vi "Dashboard Main.vi"() -> ()   [LabVIEW 2016]
uses:
  <vilib>/Utility/miscctls.llb/LVRowAndColumnTypeDef.ctl
  <vilib>/event_ctls.llb/eventvkey.ctl
  <vilib>/Rock Robotics/Network Tables/NT Read Numeric Array.vi
  <vilib>/Rock Robotics/WPI/Dashboard/WPI_DashboardLogging Global.vi
panel:
  in  "Camera Settings Right":T1={"Frame Rate"=30, "Compression"=30, "Size"=1, "DB Camera Config"=FALSE} {"Frame Rate" scale=1.0..30.0; "Compression" scale=100.0..-1.0; "Size" items=["640x480", "320x240", "160x120"]}
  in  "Camera Name Right":string(combo)="No Camera Selection"
  out "Camera Info":cluster{"Mbps LED":bool, "Mbps":dbl, "fps":dbl} {"fps" format="%#.1g"; "Mbps" format="%#.1g"}
  in  "Camera Settings":T1={"Frame Rate"=30, "Compression"=30, "Size"=1, "DB Camera Config"=FALSE} {"Frame Rate" scale=1.0..30.0; "Compression" scale=100.0..-1.0; "Size" items=["640x480", "320x240", "160x120"]}
  in  "TCP":refnum<k5>
  in  "Rec Mode":enum32{"Stop", "Record", "Playback"}(radio)
  out "Robot IP":string
  out "Image Message":string="Timeout in Camera Communications"
  in  "Dashboard Tab":T2(tab)
  out "Distance (ft)":dbl(slide) scale=1.0..16.25
  in  "Select Auto":string(combo)="Select Autonomous ..."
  out "NT Connection":bool
  out "MotorChart R":cluster{"Numeric":dbl, "Numeric":dbl}(graph)
  out "MotorChart L":cluster{"Numeric":dbl, "Numeric":dbl}(graph)
  out "MotorSliders R":cluster{"MotorSlide1":dbl, "MotorSlide2":dbl} {"MotorSlide2" scale=-1.0..1.0 scale format="%#_2e"; "MotorSlide1" scale=-1.0..1.0 scale format="%#_2e"}
  out "MotorSliders L":cluster{"MotorSlide1":dbl, "MotorSlide2":dbl} {"MotorSlide2" scale=-1.0..1.0 scale format="%#_2e"; "MotorSlide1" scale=-1.0..1.0 scale format="%#_2e"}
  out "JS1 Z":dbl(slide) scale=-1.0..1.0 scale format="%#_2e"
  out "JS1 Graph":cluster{"X":dbl, "Y":dbl}[](graph)
  out "JS1 Buttons":T3
  out "JS2 Z":dbl(slide) scale=-1.0..1.0 scale format="%#_2e"
  out "JS2 Graph":cluster{"X":dbl, "Y":dbl}[](graph)
  out "JS2 Buttons":T3
  out "Mode":T4(ring)=enum."Auto Disabled"
  out "Camera Image Right":T5(plugin-control)
  in  "DB/String 9":string
  in  "DB/String 8":string
  in  "DB/String 7":string
  in  "DB/String 6":string
  in  "DB/String 5":string
  in  "DB/String 4":string
  in  "DB/String 3":string
  in  "DB/String 2":string
  in  "DB/String 1":string
  in  "DB/String 0":string
  in  "DB/Slider 0":dbl(slide) scale=0.0..5.0
  in  "DB/Slider 1":dbl(slide) scale=0.0..5.0
  in  "DB/Slider 2":dbl(slide) scale=0.0..5.0
  in  "DB/Slider 3":dbl(slide) scale=0.0..5.0
  out "DB/LED 3":bool
  out "DB/LED 2":bool
  out "DB/LED 1":bool
  out "DB/LED 0":bool
  in  "DB/Button 3":bool
  in  "DB/Button 2":bool
  in  "DB/Button 1":bool
  in  "DB/Button 0":bool caption="New Name"
  in  "Test Slider":dbl(slide) scale=0.0..100.0 scale format="%#_3g"
  in  "On/Off":bool caption="Solenoid"
  in  "Test Name":u16(ring) items=["Select the test to run..."]
  in  "Test Tree":string(tree)
  in  "Motor":cluster{"Value":dbl, "Enable":bool} {"Value" scale=-1.0..1.0 scale format="%#_3g"}
  out "Progress":T6 {"Test Progress" scale=0.0..100.0}
  in  "Rev/Fwd":cluster{"Forward":bool, "Reverse":bool}
  in  "Test Ring":u16(ring) items=["Monochrome", "Color"]
  out "Cmd Status":string
  in  "Execute Command":bool
  in  "Command Params":string[][](table)
  in  "Command Selection":i32(listbox)
  in  "CheckList":i32(listbox)
  out "Tree":string(tree)
  out "Camera Image":T5(plugin-control)
  out "Background":bool
  in  "Camera Name":string(combo)="No Camera Selection"
  # "HW"
  # "HW"
  # "Joysticks"
  # "Drive Motors"
  # "Front"
  # "Right"
  # "Left"
  # "Back"
  # "This tab is a great place for autonomous settings and robot-specific values.\nPlace controls and indicators inside this tab and match name to\nDashboard Variables on robot. You can also delete this comment."
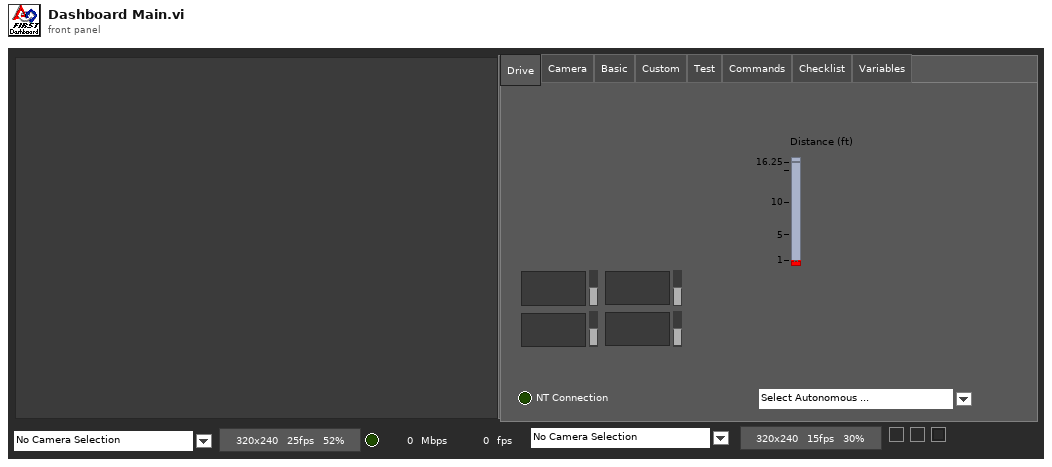
[diagram p1: front panel]
types:
  T1 = cluster{"Frame Rate":i32, "Compression":i32, "Size":u16, "DB Camera Config":bool}
  T2 = enum32{"Drive", "Camera", "Basic", "Custom", "Test", "Commands", "Checklist", "Variables"}
  T3 = cluster{bool, bool, bool, bool, bool, bool, bool, bool, bool, bool, bool, bool}
  T4 = enum8{"Tele-Op Disabled", "Tele-Op Enabled", "Auto Disabled", "Auto Enabled", "Test Disabled", "Test Enabled", "Disconnected", "No Code", "E-Stop"}
  T5 = typedef "IMAQ Image.ctl" = refnum<image>
  T6 = cluster{"Test Progress":u8, "Test Progress Text":string}
  T7 = typedef "Image Type" = u32
  T8 = cluster{"IDs":cluster{"RPC field ID":u16, "Unique ID":u16}, "String":string}
  T9 = enum32{"Drive", "Basic", "Custom", "Test", "Checklist", "Variables"}
  T10 = cluster{"Error Strings":string, "Disable Counts":cluster{u16, u16}, "Rail Faults":cluster{u16, u16, u16}, "Robot IP":string, "DB Mode":u8, "Event Info":cluster{"Name":string, "Type":u8, "Number":u16, "Replay":u8}}
  T11 = cluster{"Storage":cluster{"Disk Free":u64, "RAM Block":u32, "RAM free":u32}, "CPU Utilization":cluster{"CPU % ISR":sgl, "CPU % Time Crit":sgl, "CPU % Timed Str":sgl, "CPU % High":sgl, "CPU % Above":sgl, "CPU % Normal":sgl, "CPU % Low":sgl}, "CAN":cluster{"% Bus Utilization":sgl, "Bus Off Cnt":u32, "TX_FIFO Full Cnt":u32, "Receive Error Cnt":u8, "Transmit Error Cnt":u8}, "HID":cluster{"HID Outputs":u32, "Rumble Low":u16, "Rumble High":u16}[]}
  T12 = cluster{"Status bits":cluster{"Test Mode":bool, "Autonomous":bool, "Enabled":bool, "Code Start":bool, "Brownout":bool, "Reserved 2":bool, "Reserved 3":bool, "E-Stop":bool}, "Code Trace":cluster{"Disabled":bool, "TeleOp":bool, "Auto":bool, "Test":bool}, "Controller Type":enum16{"unknown", "cRIO", "roboRio"}, "Code?":enum16{"unknown", "noCode", "code"}, "Battery V":dbl}
  T13 = cluster{"Control Bits":cluster{"TestMode":bool, "Autonomous":bool, "Enabled":bool, "FMS Present":bool, bool, bool, bool, "E-Stop":bool}, "Team Station ":u8, "Countdown":sgl, "Joystick Values":cluster{"Axes":dbl[], "Buttons":bool[], "POVs":i16[]}[]}
  T14 = cluster{"Axes":dbl[], "Buttons":bool[], "POVs":i16[]}[]
  T15 = cluster{"Axes":dbl[], "Buttons":bool[], "POVs":i16[]}
  T16 = cluster{"Buttons[0]":bool, "Buttons[1]":bool, "Buttons[2]":bool, "Buttons[3]":bool, "Buttons[4]":bool, "Buttons[5]":bool, "Buttons[6]":bool, "Buttons[7]":bool, "Buttons[8]":bool, "Buttons[9]":bool, "Buttons[10]":bool, "Buttons[11]":bool}
  T17 = cluster{"Camera Image":refnum<vi>, "Dashboard Tab":refnum<vi>, "Background":refnum<vi>, "Rec Mode":refnum<vi>, "Test Slider":refnum<vi>, "On/Off ":refnum<vi>, "Test Ring":refnum<vi>, "Rev/Fwd":refnum<vi>, "Test Name":refnum<vi>, "Motor":refnum<vi>, "Progress":refnum<vi>, "CheckList":refnum<vi>, "Tree":refnum<vi>, "Test Tree":refnum<vi>, "Command Params":refnum<vi>, "Command Selection":refnum<vi>, "Execute Command":refnum<vi>, "Cmd Status":refnum<vi>, "Camera Settings":refnum<vi>, "Camera Name":refnum<vi>, "Camera Info":refnum<vi>, "Camera Settings Right":refnum<vi>, "Camera Name Right":refnum<vi>, "Camera Image Right":refnum<vi>}
  T18 = cluster{"Operation":enum16{"Update", "Clear"}, "Color Box":u32}[]
  T19 = typedef "eventvkey.ctl" = enum16{"ASCII", "Enter", "Return", "Shift", "Ctrl", "Alt", "Cmd", "Opt", "Caps", "NumLock", "Clear", "Break", "Up", "Down", "Left", "Right", "Insert", "Delete", "Home", "End", "PageUp", "PageDown", "Escape", "Help", "Pause", "ScrollLock", "F1", "F2", "F3", "F4", "F5", "F6", "F7", "F8", "F9", "F10", "F11", "F12", "F13", "F14", "F15", "F16", "F17", "F18", "F19", "F20", "F21", "F22", "F23", "F24", "Play", "VolumeUp", "VolumeDown", "Mute", "Two Byte Char"}
  T20 = cluster{"Image Size":bool, "Image Type":bool, "Pixel Value":bool, "ROI Information":bool, "Zoom Factor":bool}
  T21 = cluster{"Operation":enum16{"Update", "Clear"}, "Color Box":u32}
  T22 = typedef "LVRowAndColumnTypeDef.ctl" = cluster{"Row":i32, "Column":i32}
  T23 = cluster{"Shift":bool, "Ctrl":bool, "Alt":bool, "Cmd":bool, "Opt":bool}
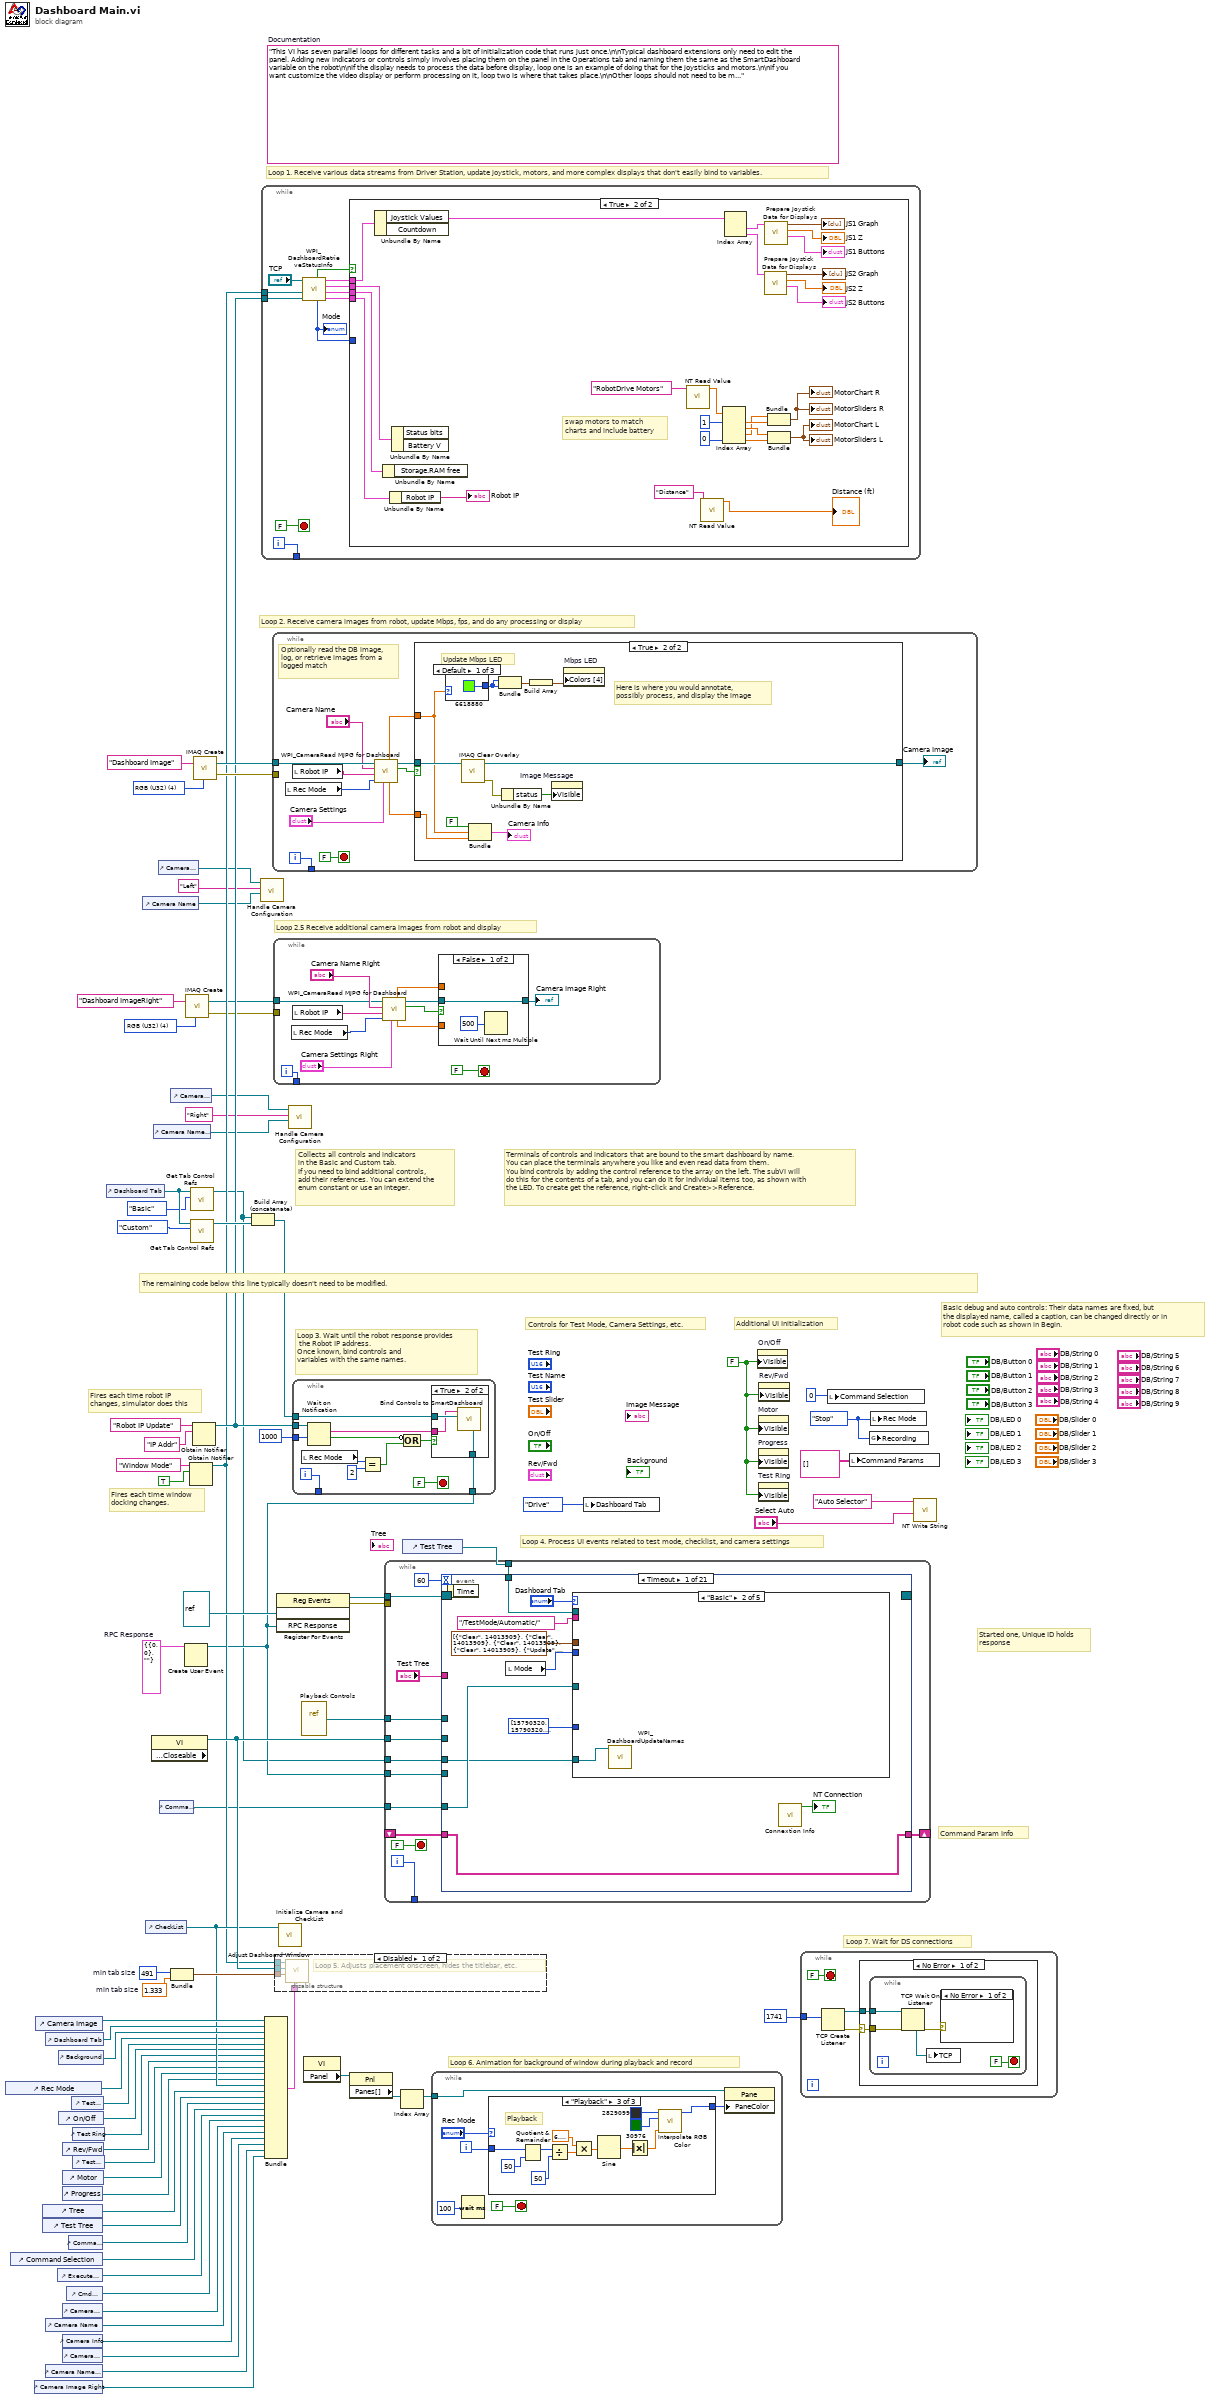
[diagram p0: block diagram]
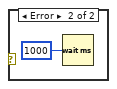
[diagram p4: hidden frame]
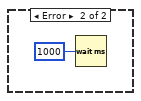
[diagram p5: hidden frame]
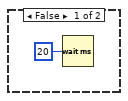
[diagram p6: hidden frame]
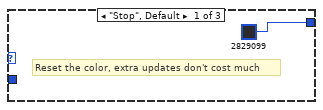
[diagram p7: hidden frame]
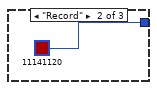
[diagram p8: hidden frame]
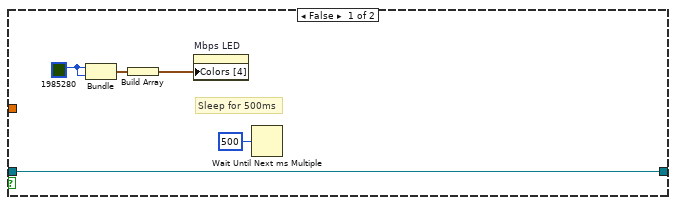
[diagram p10: hidden frame]
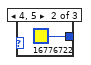
[diagram p11: hidden frame]
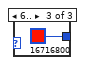
[diagram p12: hidden frame]
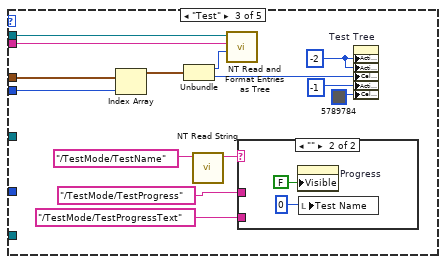
[diagram p14: hidden frame]
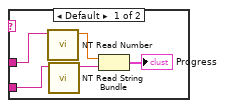
[diagram p15: hidden frame]
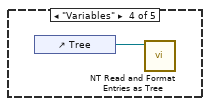
[diagram p16: hidden frame]
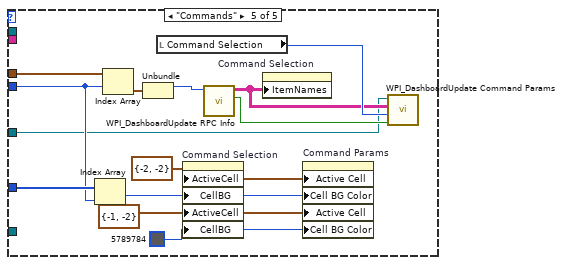
[diagram p17: hidden frame]
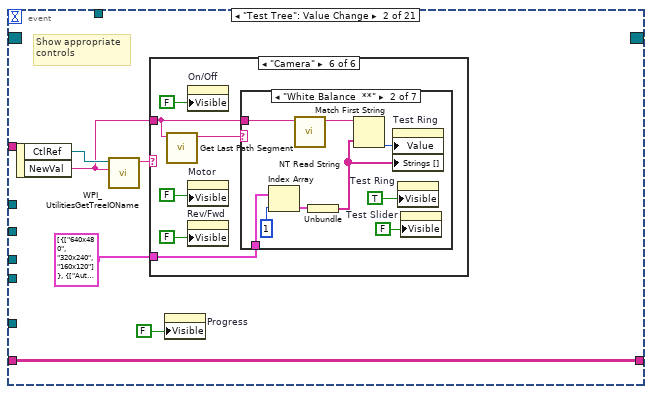
[diagram p18: hidden frame]
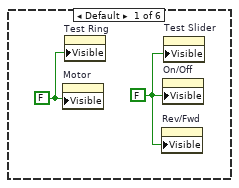
[diagram p19: hidden frame]
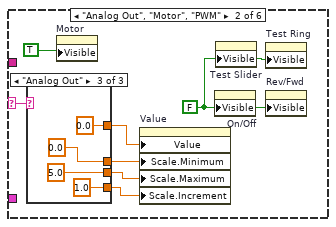
[diagram p20: hidden frame]
diagram:
  w10 = T7 4 items=["Grayscale (U8)", "Grayscale (I16)", "Grayscale (SGL)", "Complex (CSG)", "RGB (U32)", "HSL (U32)", "RGB (U64)"] ("Image Type")
  w26 = T8 {"IDs"={"RPC field ID"=0, "Unique ID"=0}, "String"=""}  # RPC Response
  w51 = 491  # min tab size
  w50 = 1.333  # min tab size
  w58 = enum32{"Stop", "Record", "Playback"}."Stop" ("Rec Mode")
  w33 = FALSE ("Visible")
  (unwired) "This VI has seven parallel loops for different tasks and a bit of initialization code that runs just once.\n\nTypical dashboard extensions only need to edit the panel. Adding new indicators or controls simply involves placing them on the panel in the Operations tab and naming them the same as the SmartDashboard variable on the robot\n\nIf the display needs to process the data before display, loop one is an example of doing that for the joysticks and motors.\n\nIf you want customize the video display or perform processing on it, loop two is where that takes place.\n\nOther loops should not need to be modified. They are pretty standard, and document the task they perform."  # Documentation
  w75 = T7 4 items=["Grayscale (U8)", "Grayscale (I16)", "Grayscale (SGL)", "Complex (CSG)", "RGB (U32)", "HSL (U32)", "RGB (U64)"] ("Image Type")
  # "Loop 2.5 Receive additional camera images from robot and display"
  # "Command Param Info"
  # "Started one, Unique ID holds\nresponse"
  # "Loop 7. Wait for DS connections"
  # "Basic debug and auto controls: Their data names are fixed, but\nthe displayed name, called a caption, can be changed directly or in\nrobot code such as shown in Begin."
  # "Controls for Test Mode, Camera Settings, etc."
  # "Additional UI Initialization"
  # "Loop 6. Animation for background of window during playback and record"
  # "Fires each time robot IP\nchanges, simulator does this"
  # "Fires each time window\ndocking changes."
  # "Collects all controls and indicators\nin the Basic and Custom tab.\nIf you need to bind additional controls,\nadd their references. You can extend the\nenum constant or use an integer."
  # "The remaining code below this line typically doesn't need to be modified."
  # "Loop 4. Process UI events related to test mode, checklist, and camera settings"
  # "Terminals of controls and indicators that are bound to the smart dashboard by name.\nYou can place the terminals anywhere you like and even read data from them.\nYou bind controls by adding the control reference to the array on the left. The subVI will\ndo this for the contents of a tab, and you can do it for individual items too, as shown with\nthe LED. To create get the reference, right-click and Create>>Reference."
  # "Loop 3. Wait until the robot response provides\n the Robot IP address.\nOnce known, bind controls and\nvariables with the same names."
  # "Loop 1. Receive various data streams from Driver Station, update joystick, motors, and more complex displays that don't easily bind to variables."
  # "Loop 2. Receive camera images from robot, update Mbps, fps, and do any processing or display"
  n1 = control-ref of="Rec Mode"() -> (w39:refnum<vi>)
  n2 = control-ref of="Command Selection"() -> (w25:refnum<vi>)
  n3 = control-ref of="Camera Image Right"() -> (w1:refnum<vi>)
  n4 = control-ref of="Camera Image"() -> (w53:refnum<vi>)
  n5 = control-ref of="Tree"() -> (w43:refnum<vi>)
  n6 = control-ref of="Test Tree"() -> (w42:refnum<vi>)
  n7 = control-ref of="Dashboard Tab"() -> (w52:refnum<vi>)
  n8 = control-ref of="Camera Name"() -> (w16:refnum<vi>)
  n9 = control-ref of="Camera Name Right"() -> (w2:refnum<vi>)
  n10 = control-ref of="Execute Command"() -> (w27:refnum<vi>)
  n11 = control-ref of="Background"() -> (w48:refnum<vi>)
  n12 = control-ref of="On/Off"() -> (w37:refnum<vi>)
  n13 = control-ref of="Progress"() -> (w34:refnum<vi>)
  n14 = control-ref of="Camera Settings"() -> (w17:refnum<vi>)
  n15 = control-ref of="Camera Info"() -> (w15:refnum<vi>)
  n16 = control-ref of="Camera Settings Right"() -> (w3:refnum<vi>)
  n17 = control-ref of="Rev/Fwd"() -> (w35:refnum<vi>)
  n18 = control-ref of="Motor"() -> (w40:refnum<vi>)
  n19 = control-ref of="Cmd Status"() -> (w21:refnum<vi>)
  n20 = control-ref of="Command Params"() -> (w28:refnum<vi>)
  n21 = control-ref of="Test Slider"() -> (w38:refnum<vi>)
  n22 = control-ref of="Test Ring"() -> (w36:refnum<vi>)
  n23 = control-ref of="Test Name"() -> (w41:refnum<vi>)
  n24 = control-ref of="Dashboard Tab"() -> (w56:refnum<vi>)
  n25 = control-ref of="Camera Name"() -> (w18:refnum<vi>)
  n26 = control-ref of="CheckList"() -> (w44:refnum<vi>)
  n27 = property class="VI" props=["Front Panel.Closeable"]() -> (reference out=w57:refnum<vi>)  [unwired: 2 in, 2 out]
  n28 = control-ref of="Camera Name Right"() -> (w6:refnum<vi>)
  n29 = control-ref of="Camera Settings"() -> (w19:refnum<vi>)
  n30 = control-ref of="Command Params"() -> (w20:refnum<vi>)
  n31 = control-ref of="Camera Settings Right"() -> (w7:refnum<vi>)
  n32 = Bundle("min tab size"=w51, "min tab size"=w50) -> (w49:cluster{"min tab size":i32, "min tab size":dbl})  [unwired: 1 in]
  n33 = Create User Event(user event datatype=w26) -> (user event=w22:refnum<user-event>)  [unwired: 1 in, 1 out]
  n34 = call "IMAQ Create"("Image Name"="Dashboard ImageRight", "Image Type"=w10) -> ("New Image"=w9:T5, "error out"=w8:errorcluster)  [unwired: 2 in, 1 out]
  n35 = Obtain Notifier(name (unnamed)="Window Mode", notification data type=TRUE) -> (notifier out=w31:refnum<notifier>)  [unwired: 2 in, 2 out]
  n36 = call <vilib>:"Get Tab Control Refs.vi"("Page Index"=T9."Basic" ("Dashboard Tab"), "TabControl in"=w56) -> ("ControlsOnPage"=w14:refnum<vi>[])  [unwired: 9 in]
  n37 = call <vilib>:"Get Tab Control Refs.vi"("Page Index"=T9."Custom" ("Dashboard Tab"), "TabControl in"=w56) -> ("ControlsOnPage"=w55:refnum<vi>[])  [unwired: 9 in]
  n38 = Obtain Notifier(name (unnamed)="Robot IP Update", notification data type="IP Addr" ("name (unnamed)")) -> (notifier out=w32:refnum<notifier>)  [unwired: 2 in, 2 out]
  n39 = call "IMAQ Create"("Image Name"="Dashboard Image", "Image Type"=w75) -> ("New Image"=w73:T5, "error out"=w72:errorcluster)  [unwired: 2 in, 1 out]
  n40 = Build Array (concatenate)(w14, w55) -> (w54:refnum<vi>[])
  n41 = call "Handle Camera Configuration.vi"("CameraNameRef"=w18, "Camera File Name"="Left", "ClusterRef"=w19) -> ()  [unwired: 9 in]
  n42 = while {
    tunnel: [w85] -> _
    tunnel: w32 -> [w79]
    tunnel: w31 -> [w76]
    i -> [w85]
    stop <- FALSE stop-if-true
    n43 = call <vilib>:"WPI_DashboardRetrieveStatusInfo.vi"("Binding Refnum"=w79, "Window Mode Notifier"=w76, "TCP Cnx"="TCP") -> ("Power and Errors"=w80:T10, "Robot Metrics"=w83:T11, "Status Info"=w84:T12, "Control Info"=w81:T13, "Robot Mode"=w78:T4, "Process?"=w82:bool)  [unwired: 3 in]
    "Mode" <- w78
    n44 = case shown="True" w82 {
      tunnel: w84 -> [_ w113]
      tunnel: w83 -> [_ w112]
      tunnel: w81 -> [_ w111]
      tunnel: w80 -> [_ w110]
      tunnel: w78 -> [_ _]
      frame False {
        n45 = Wait (ms)(milliseconds to wait=u32 20) -> ()  [unwired: 1 out]
      }
      frame True {
        # "swap motors to match\ncharts and include battery"
        n46 = Unbundle By Name(w111) -> ("Joystick Values"=w101:T14)  [unwired: 1 out]
        n47 = Unbundle By Name(w112) -> ()  [unwired: 1 out]
        n48 = Unbundle By Name(w110) -> ("Robot IP"=→"Robot IP":string)
        n49 = Unbundle By Name(w113) -> ()  [unwired: 2 out]
        n50 = call-poly <vilib>:"NT Read Value.vi"("Name"="RobotDrive Motors") -> ("Numeric Array"=w91:dbl[])  [unwired: 9 in, 1 out]
        n51 = call-poly <vilib>:"NT Read Value.vi"("Name"="Distance") -> ("Numeric"=→"Distance (ft)":dbl)  [unwired: 9 in, 1 out]
        n52 = Index Array(array=w91, index #1=1, index #4=0) -> (element #1=w105:dbl, element #2=w106:dbl, element #3=w104:dbl, element #4=w109:dbl)  [unwired: 2 in]
        n53 = Index Array(array=w101) -> (element #1=w100:T15, element #2=w96:T15)  [unwired: 2 in]
        n54 = call "Prepare Joystick Data for Displays.vi"("Joystick Values"=w96) -> ("Buttons"=→"JS2 Buttons":T16, "Z Axis"=→"JS2 Z":dbl, "Cartesian Data"=→"JS2 Graph":cluster{"X axis":dbl, "X axis":dbl}[])  [unwired: 8 in]
        n55 = call "Prepare Joystick Data for Displays.vi"("Joystick Values"=w100) -> ("Buttons"=→"JS1 Buttons":T16, "Z Axis"=→"JS1 Z":dbl, "Cartesian Data"=→"JS1 Graph":cluster{"X axis":dbl, "X axis":dbl}[])  [unwired: 8 in]
        n56 = Bundle("Numeric"=w104, "Numeric"=w105) -> (→"MotorChart R" →"MotorSliders R":cluster{"Numeric":dbl, "Numeric":dbl})  [unwired: 1 in]
        n57 = Bundle("Numeric"=w106, "Numeric"=w109) -> (→"MotorChart L" →"MotorSliders L":cluster{"Numeric":dbl, "Numeric":dbl})  [unwired: 1 in]
      }
    }
  }
  n58 = Bundle("Camera Image"=w53, "Dashboard Tab"=w52, "Background"=w48, "Rec Mode"=w39, "Test Slider"=w38, "On/Off"=w37, "Test Ring"=w36, "Rev/Fwd"=w35, "Test Name"=w41, "Motor"=w40, "Progress"=w34, "CheckList"=w44, "Tree"=w43, "Test Tree"=w42, "Command Params"=w28, "Command Selection"=w25, "Execute Command"=w27, "Cmd Status"=w21, "Camera Settings"=w17, "Camera Name"=w16, "Camera Info"=w15, "Camera Settings Right"=w3, "Camera Name Right"=w2, "Camera Image Right"=w1) -> (w45:T17)  [unwired: 1 in]
  n59 = while {
    tunnel: w73 -> [w123]
    tunnel: w72 -> [_]
    tunnel: [w124] -> _
    i -> [w124]
    stop <- FALSE stop-if-true
    # "Optionally read the DB image,\nlog, or retrieve images from a\nlogged match"
    n60 = local read "Rec Mode"() -> (w119:enum32{"Stop", "Record", "Playback"})
    n61 = local read "Robot IP"() -> (w118:string)
    n62 = call <vilib>:"WPI_CameraRead MJPG for Dashboard.vi"("Camera Settings"="Camera Settings", "Rec Mode"=w119, "Robot IP"=w118, "Camera Name"="Camera Name", "Refnum in"=w123) -> ("Active"=w121:bool, "Refnum out"=w122:T5, "FPS"=w120:dbl, "Bandwidth (Mbps)"=w117:dbl)  [unwired: 3 in]
    n63 = case shown="True" w121 {
      tunnel: w122 -> [w126 w137]
      tunnel: w117 -> [_ w134]
      tunnel: w120 -> [_ w135]
      tunnel: [w126 w131] -> w114
      frame False {
        w128 = u32 1985280 ("Color Box")
        # "Sleep for 500ms"
        n64 = Bundle("Color Box"=w128, "Color Box"=w128) -> (w129:cluster{"Color Box":u32, "Color Box":u32})  [unwired: 1 out]
        n65 = Build Array(w129) -> (w127:cluster{"Color Box":u32, "Color Box":u32}[])
        n66 = property on="Mbps LED" class="Bool (strict)"("Colors [4]"=w127) -> ()  [unwired: 2 in, 2 out]
        n67 = Wait Until Next ms Multiple(millisecond multiple=u32 500) -> ()  [unwired: 1 out]
      }
      frame True {
        # "Here is where you would annotate,\npossibly process, and display the image"
        # "Update Mbps LED"
        n68 = case shown="Default" w134 {
          tunnel: [u32 6618880 ("Color Box") u32 16776722 ("Color Box") u32 16716800 ("Color Box")] -> w138
          frame Default {
          }
          frame 4, 5 {
          }
          frame 6.. {
          }
        }
        n69 = call "IMAQ Clear Overlay"("Image"=w137) -> ("error out"=w140:errorcluster, "Image Out"=w131:T5)  [unwired: 2 in, 7 out]
        n70 = Bundle(FALSE, "Bandwidth (Mbps)"=w134, "FPS"=w135) -> (→"Camera Info":cluster{bool, "Bandwidth (Mbps)":dbl, "FPS":dbl})  [unwired: 1 in]
        n71 = Bundle("Color Box"=w138, "Color Box"=w138) -> (w139:cluster{"Color Box":u32, "Color Box":u32})  [unwired: 1 out]
        n72 = Unbundle By Name(w140) -> ("status"=w141:bool)
        n73 = Build Array(w139) -> (w136:cluster{"Color Box":u32, "Color Box":u32}[])
        n74 = property on="Image Message" class="Str"("Visible"=w141) -> ()  [unwired: 2 in, 2 out]
        n75 = property on="Mbps LED" class="Bool (strict)"("Colors [4]"=w136) -> ()  [unwired: 2 in, 2 out]
      }
    }
    "Camera Image" <- w114
  }
  n76 = while {
    tunnel: w9 -> [w155]
    tunnel: w8 -> [_]
    tunnel: [w149] -> _
    i -> [w149]
    stop <- FALSE stop-if-true
    n77 = local read "Rec Mode"() -> (w153:enum32{"Stop", "Record", "Playback"})
    n78 = local read "Robot IP"() -> (w154:string)
    n79 = call <vilib>:"WPI_CameraRead MJPG for Dashboard.vi"("Camera Settings"="Camera Settings Right", "Rec Mode"=w153, "Robot IP"=w154, "Camera Name"="Camera Name Right", "Refnum in"=w155) -> ("Active"=w148:bool, "Refnum out"=w151:T5, "FPS"=w146:dbl, "Bandwidth (Mbps)"=w147:dbl)  [unwired: 3 in]
    n80 = case shown="False" w148 {
      tunnel: w151 -> [w157 w159]
      tunnel: w147 -> [_ _]
      tunnel: w146 -> [_ _]
      tunnel: [w157 w159] -> w145
      frame False {
        n81 = Wait Until Next ms Multiple(millisecond multiple=u32 500) -> ()  [unwired: 1 out]
      }
      frame True {
      }
    }
    "Camera Image Right" <- w145
  }
  n82 = disable-structure shown="Disabled" {
    disable-tunnel: w57 -> [w163 _]
    disable-tunnel: w49 -> [w162 _]
    disable-tunnel: w45 -> [w161 _]
    disable-tunnel: w31 -> [w160 _]
    frame Disabled {
      # "Loop 5. Adjusts placement onscreen, hides the titlebar, etc."
      n83 = call "Adjust Dashboard Window.vi"("Sizing Refnums"=w161, "Size Constraints"=w162, "VI"=w163, "WIn Mode"=w160) -> ()  [unwired: 8 in]
    }
    frame Enabled {
    }
  }
  n84 = register-events(refnum<vi> refnum, w22) -> (reference out=w62:refnum<event-registration>, error out=w61:errorcluster)  [unwired: 2 in]
  n85 = call "Initialize Camera and CheckList.vi"("ListBox in"=w44) -> ()  [unwired: 11 in]
  n86 = call "Handle Camera Configuration.vi"("CameraNameRef"=w6, "Camera File Name"="Right", "ClusterRef"=w7) -> ()  [unwired: 9 in]
  n87 = while {
    tunnel: w54 -> [w175]
    tunnel: w32 -> [w173]
    tunnel: [w171] -> _
    tunnel: u32 1000 ("milliseconds to wait") -> [w170]
    tunnel: w22 -> [w164]
    i -> [w171]
    stop <- FALSE stop-if-true
    n88 = local read "Rec Mode"() -> (w166:enum32{"Stop", "Record", "Playback"})
    n89 = Wait on Notification(notifier=w173, timeout in ms (-1)=w170) -> (notification=w172:string, timed out?=w168:bool)  [unwired: 2 in, 2 out]
    n90 = Equal?(x=w166, y=u16 2 ("Rec Mode")) -> (x = y?=w167:bool)
    n91 = Compound Arithmetic op=OR(invert w168, w167) -> (w169:bool)
    n92 = case shown="True" w169 {
      tunnel: w175 -> [_ w178]
      tunnel: w172 -> [_ w177]
      tunnel: w164 -> [_ w176]
      frame False {
      }
      frame True {
        n93 = call <vilib>:"Bind Controls to SmartDashboard.vi"("RPC ref"=w176, "Bound Control Refs"=w178, "Server IP Address"=w177) -> ()  [unwired: 9 in]
      }
    }
  }
  n94 = vi-ref "Playback Controls.vi"() -> (w63:refnum<vi>)
  n95 = property class="VI"() -> ("Panel"=w65:refnum<vi>)  [unwired: 2 in, 2 out]
  n96 = property class="Pnl"(reference=w65) -> ("Panes[]"=w66:refnum<vi>[])  [unwired: 1 in, 2 out]
  n97 = Index Array(array=w66) -> (element=w64:refnum<vi>)  [unwired: 1 in]
  n98 = control-ref of="Test Tree"() -> (w67:refnum<vi>)
  n99 = while {
    tunnel: [w188] -> _
    tunnel: w67 -> [w187]
    tunnel: w63 -> [w186]
    tunnel: w62 -> [w185]
    tunnel: w61 -> [_]
    tunnel: w57 -> [w184]
    tunnel: w22 -> [w183]
    tunnel: w20 -> [w182]
    shift-right: [w181] -> _
    shift-left: _ -> [w180]
    tunnel: w14 -> [w179]
    i -> [w188]
    stop <- FALSE stop-if-true
    n100 = event shown="[0] Timeout" {
      selector: w185 -> [_ _ _ _ _ _ _ _ _ _ _ _ _ _ _ _ _ _ _ _ _]
      dyn-events: [_ _ _ _ _ _ _ _ _ _ _ _ _ _ _ _ w444 _ _ _ _] -> _
      timeout: u32 60 ("milliseconds to wait") -> [_ _ _ _ _ _ _ _ _ _ _ _ _ _ _ _ _ _ _ _ _]
      tunnel: w187 -> [w200 _ _ _ _ _ _ _ _ _ _ _ _ _ _ _ _ _ _ _ _]
      tunnel: "Test Tree" -> [_ _ _ _ _ _ _ _ _ _ _ w411 w419 w421 w425 w433 _ _ _ _ _]
      tunnel: w186 -> [_ _ _ _ _ _ _ _ _ _ _ _ _ _ _ _ w446 _ w464 _ _]
      tunnel: w184 -> [_ _ _ _ _ _ _ _ _ _ _ _ _ _ _ _ w442 _ _ _ _]
      tunnel: w183 -> [_ _ _ _ _ _ _ _ _ _ _ _ _ _ _ _ w438 _ _ _ _]
      tunnel: w182 -> [w195 _ _ _ _ _ w362 _ _ _ _ _ _ _ _ _ _ _ _ _ _]
      tunnel: [w194 w239 w341 w346 w355 w359 w360 w369 w379 w386 w398 w410 w417 w420 w424 w432 w437 w459 w461 w465 w476] -> w181
      tunnel: w180 -> [w194 w239 w341 w346 w355 w359 w360 _ _ w386 w398 w410 w417 w420 w424 w432 w437 w459 w461 w465 w476]
      tunnel: w179 -> [w192 _ _ _ _ _ _ _ _ _ _ _ _ _ _ _ _ _ _ _ _]
      event Timeout {
        n101 = event-data() -> ()  [unwired: 1 in, 1 out]
        n102 = local read "Mode"() -> (w197:T4)
        n103 = case shown="\"Basic\"" "Dashboard Tab" {
          tunnel: w200 -> [_ _ w216 _ _]
          tunnel: "/TestMode/Automatic/" ("Name Pattern") -> [_ _ w215 _ _]
          tunnel: T18 [{"Operation"=enum."Clear", "Color Box"=14013909}, {"Operation"=enum."Clear", "Color Box"=14013909}, {"Operation"=enum."Clear", "Color Box"=14013909}, {"Operation"=enum."Clear", "Color Box"=14013909}, {"Operation"=enum."Update", "Color Box"=14013909}, {"Operation"=enum."Update", "Color Box"=16777215}, {"Operation"=enum."Clear", "Color Box"=14013909}, {"Operation"=enum."Clear", "Color Box"=14013909}, {"Operation"=enum."Clear", "Color Box"=14013909}] -> [_ _ w208 _ w232]
          tunnel: w197 -> [_ _ w207 _ w231]
          tunnel: u32[] [15790320, 15790320, 15790320, 15790320, 16777215, 16777215, 15790320, 15790320, 15790320] -> [_ _ _ _ w237]
          tunnel: w195 -> [_ _ _ _ w225]
          tunnel: w192 -> [_ w202 _ _ _]
          frame "Custom", Default {
          }
          frame "Basic" {
            n104 = call <vilib>:"WPI_DashboardUpdateNames.vi"("Controls on Tab"=w202) -> ()  [unwired: 11 in]
          }
          frame "Test" {
            w214 = -2 ("Active Item:Row Number")
            n105 = Index Array(array=w208, index=w207) -> (element=w209:T21)
            n106 = Unbundle(w209) -> ("Operation"=w210:enum16{"Update", "Clear"}, "Color Box"=w211:u32)
            n107 = call <vilib>:"NT Read String.vi"("Name"="/TestMode/TestName") -> ("String"=w205:string)  [unwired: 9 in, 1 out]
            n108 = call <vilib>:"NT Read and Format Entries as Tree.vi"("Operation"=w210, "Name Pattern"=w215, "Tree Refnum"=w216) -> ()  [unwired: 7 in, 2 out]
            n109 = case shown="\"\"" w205 {
              tunnel: "/TestMode/TestProgress" ("Name") -> [w218 _]
              tunnel: "/TestMode/TestProgressText" ("Name") -> [w217 _]
              frame Default {
                n110 = call <vilib>:"NT Read Number.vi"("Name"=w218) -> ("Numeric"=w219:dbl)  [unwired: 9 in, 1 out]
                n111 = call <vilib>:"NT Read String.vi"("Name"=w217) -> ("String"=w220:string)  [unwired: 9 in, 1 out]
                n112 = Bundle("Numeric"=w219, "String"=w220) -> (→"Progress":cluster{"Numeric":dbl, "String":string})  [unwired: 1 in]
              }
              frame "" {
                n113 = property on="Progress" class="Clust (strict)"("Visible"=FALSE) -> ()  [unwired: 2 in, 2 out]
                n114 = local write "Test Name"(u16 0) -> ()
              }
            }
            n115 = property on="Test Tree" class="Tree (strict)"("Active Item Row Number"=w214, "ActiveColNum"=w214, "CellBG"=w211, "Active Item Row Number"=-1 ("Active Item:Row Number"), "CellBG"=u32 5789784 ("Color Box")) -> ()  [unwired: 2 in, 2 out]
          }
          frame "Variables" {
            n116 = control-ref of="Tree"() -> (w224:refnum<vi>)
            n117 = call <vilib>:"NT Read and Format Entries as Tree.vi"("Tree Refnum"=w224) -> ()  [unwired: 9 in, 2 out]
          }
          frame "Commands" {
            w233 = u32 5789784 ("Color Box")
            w234 = T22 {"Row"=-1, "Column"=-2} ("Active Cell:Active Cell")
            w236 = T22 {"Row"=-2, "Column"=-2} ("Active Cell:Active Cell")
            n118 = Index Array(array=w237, index=w231) -> (element=w235:u32)
            n119 = Index Array(array=w232, index=w231) -> (element=w230:T21)
            n120 = Unbundle(w230) -> ("Operation"=w229:enum16{"Update", "Clear"})  [unwired: 1 out]
            n121 = local read "Command Selection"() -> (w228:i32)
            n122 = property on="Command Selection" class="MCListbox (strict)"("ActiveCell"=w236, "CellBG"=w235, "ActiveCell"=w234, "CellBG"=w233) -> ()  [unwired: 2 in, 2 out]
            n123 = call <vilib>:"WPI_DashboardUpdate RPC Info.vi"("Operation"=w229) -> ("update"=w227:bool, "commands"=w226:string[][])  [unwired: 9 in]
            n124 = property on="Command Selection" class="MCListbox (strict)"("ItemNames"=w226) -> ()  [unwired: 2 in, 2 out]
            n125 = property on="Command Params" class="Tbl (strict)"("Active Cell"=w236, "Cell BG Color"=w235, "Active Cell"=w234, "Cell BG Color"=w233) -> ()  [unwired: 2 in, 2 out]
            n126 = call <vilib>:"WPI_DashboardUpdate Command Params.vi"("Update"=w227, "NewVal"=w228, "Commands"=w226, "Param Tbl"=w225) -> ()  [unwired: 7 in, 1 out]
          }
        }
        n127 = call <vilib>:"Connextion Info.vi"() -> ("Connected"=→"NT Connection":bool)  [unwired: 10 in, 1 out]
      }
      event "Test Tree": Value Change {
        # "Show appropriate\ncontrols"
        n128 = event-data() -> ("CtlRef"=w242:refnum<vi>, "NewVal"=w240:string)  [unwired: 1 in]
        n129 = call <vilib>:"WPI_UtilitiesGetTreeIOName.vi"("NewVal"=w240, "TreeControl in"=w242) -> ("I/O Name"=w243:string)  [unwired: 9 in]
        n130 = case shown="\"Camera\"" w243 {
          selector: w243 -> [_ w250 _ w272 w281 _]
          tunnel: w240 -> [_ _ w269 w271 _ w288]
          tunnel: cluster{string[]}[] [{["640x480", "320x240", "160x120"]}, {["Auto", "Fixed indoor", "Fixed outdoor 1", "Fixed outdoor 2", "Fixed fluorescent 1", "Fixed fluorescent 2", "Hold current"]}, {["Auto", "Flicker-free 50 Hz", "Flicker-free 60 Hz", "Hold current"]}, {["None", "Prioritize frame rate", "Prioritize image quality"]}, {["Monochrome", "Color"]}] -> [_ _ _ _ _ w287]
          frame Default {
            w245 = FALSE ("Visible")
            w244 = FALSE ("Visible")
            n131 = property on="Motor" class="Clust (strict)"("Visible"=w244) -> ()  [unwired: 2 in, 2 out]
            n132 = property on="Test Ring" class="Ring (strict)"("Visible"=w244) -> ()  [unwired: 2 in, 2 out]
            n133 = property on="Rev/Fwd" class="Clust (strict)"("Visible"=w245) -> ()  [unwired: 2 in, 2 out]
            n134 = property on="On/Off" class="Bool (strict)"("Visible"=w245) -> ()  [unwired: 2 in, 2 out]
            n135 = property on="Test Slider" class="Slide (strict)"("Visible"=w245) -> ()  [unwired: 2 in, 2 out]
          }
          frame "Analog Out", "Motor", "PWM" {
            w251 = FALSE ("Visible")
            n136 = case shown="\"Analog Out\"" w250 {
              tunnel: [1.0 ("Value") -1.0 ("Value") 0.0 ("Value")] -> w249
              tunnel: [255.0 ("Value") 1.0 ("Value") 5.0 ("Value")] -> w248
              tunnel: [128.0 ("Value") 0.0 ("Value") 0.0 ("Value")] -> w247
              tunnel: [64.0 ("Value") 0.5 ("Value") 1.0 ("Value")] -> w246
              frame "PWM" {
              }
              frame "Motor", Default {
              }
              frame "Analog Out" {
              }
            }
            n137 = property on="Motor" class="Clust (strict)"("Visible"=TRUE) -> ()  [unwired: 2 in, 2 out]
            n138 = property on="Value" class="Slide (strict)"("Value"=w247, "Scale.Minimum"=w249, "Scale.Maximum"=w248, "Scale.Increment"=w246) -> ()  [unwired: 2 in, 2 out]
            n139 = property on="On/Off" class="Bool (strict)"("Visible"=w251) -> ()  [unwired: 2 in, 2 out]
            n140 = property on="Test Slider" class="Slide (strict)"("Visible"=w251) -> ()  [unwired: 2 in, 2 out]
            n141 = property on="Test Ring" class="Ring (strict)"("Visible"=w251) -> ()  [unwired: 2 in, 2 out]
            n142 = property on="Rev/Fwd" class="Clust (strict)"("Visible"=w251) -> ()  [unwired: 2 in, 2 out]
          }
          frame "Servo" {
            w267 = FALSE ("Visible")
            n143 = call <vilib>:"NT Read Number.vi"("Name"=w269) -> ("Numeric"=w268:dbl)  [unwired: 9 in, 1 out]
            n144 = property on="Test Slider" class="Slide (strict)"("Visible"=TRUE, "Scale.Maximum"=170.0 ("Scale.Range:Maximum")) -> ()  [unwired: 2 in, 2 out]
            n145 = local write "Test Slider"(w268) -> ()
            n146 = property on="Motor" class="Clust (strict)"("Visible"=w267) -> ()  [unwired: 2 in, 2 out]
            n147 = property on="Rev/Fwd" class="Clust (strict)"("Visible"=w267) -> ()  [unwired: 2 in, 2 out]
            n148 = property on="On/Off" class="Bool (strict)"("Visible"=w267) -> ()  [unwired: 2 in, 2 out]
            n149 = property on="Test Ring" class="Ring (strict)"("Visible"=w267) -> ()  [unwired: 2 in, 2 out]
          }
          frame "Relay", "Solenoid" {
            w270 = FALSE ("Visible")
            n150 = property on="Motor" class="Clust (strict)"("Visible"=w270) -> ()  [unwired: 2 in, 2 out]
            n151 = property on="Test Slider" class="Slide (strict)"("Visible"=w270) -> ()  [unwired: 2 in, 2 out]
            n152 = Search and Replace String(input string=w271, search string="/Value  **", replace string="/Direction") -> (result string=w277:string)  [unwired: 5 in, 3 out]
            n153 = property on="Test Ring" class="Ring (strict)"("Visible"=w270) -> ()  [unwired: 2 in, 2 out]
            n154 = call <vilib>:"NT Read String.vi"("Name"=w277) -> ("String"=w275:string)  [unwired: 9 in, 1 out]
            n155 = Equal?(x="Both directions", y=w275) -> (x = y?=w273:bool)
            n156 = Not(x=w273) -> (.not. x?=w274:bool)
            n157 = property on="Rev/Fwd" class="Clust (strict)"("Visible"=w273) -> ()  [unwired: 2 in, 2 out]
            n158 = property on="On/Off" class="Bool (strict)"("Visible"=w274, "Caption.Text"=w272) -> ()  [unwired: 2 in, 2 out]
          }
          frame "Compressor", "Digital Out" {
            w280 = FALSE ("Visible")
            # "Get direction and finish"
            n159 = property on="Motor" class="Clust (strict)"("Visible"=w280) -> ()  [unwired: 2 in, 2 out]
            n160 = property on="Test Slider" class="Slide (strict)"("Visible"=w280) -> ()  [unwired: 2 in, 2 out]
            n161 = property on="Test Ring" class="Ring (strict)"("Visible"=w280) -> ()  [unwired: 2 in, 2 out]
            n162 = property on="On/Off" class="Bool (strict)"("Visible"=TRUE, "Caption.Text"=w281) -> ()  [unwired: 2 in, 2 out]
            n163 = property on="Rev/Fwd" class="Clust (strict)"("Visible"=FALSE) -> ()  [unwired: 2 in, 2 out]
          }
          frame "Camera" {
            n164 = call <vilib>:"Get Last Path Segment.vi"("String in"=w288) -> ("String out"=w289:string)  [unwired: 10 in]
            n165 = property on="On/Off" class="Bool (strict)"("Visible"=FALSE) -> ()  [unwired: 2 in, 2 out]
            n166 = property on="Motor" class="Clust (strict)"("Visible"=FALSE) -> ()  [unwired: 2 in, 2 out]
            n167 = property on="Rev/Fwd" class="Clust (strict)"("Visible"=FALSE) -> ()  [unwired: 2 in, 2 out]
            n168 = case shown="\"White Balance  **\"" w289 {
              tunnel: w288 -> [w295 w304 w313 w322 w331 _ w337]
              tunnel: w287 -> [w293 w301 w310 w319 w328 _ _]
              frame "Size  **" {
                n169 = Index Array(array=w293) -> (element=w292:cluster{string[]})  [unwired: 1 in]
                n170 = call <vilib>:"NT Read String.vi"("Name"=w295) -> ("String"=w294:string)  [unwired: 9 in, 1 out]
                n171 = Unbundle(w292) -> (w290:string[])
                n172 = Match First String(2:w290, 3:w294) -> (0:w291:i32)  [unwired: 1 out]
                n173 = property on="Test Ring" class="Ring (strict)"("Value"=w291, "Strings []"=w290) -> ()  [unwired: 2 in, 2 out]
                n174 = property on="Test Ring" class="Ring (strict)"("Visible"=TRUE) -> ()  [unwired: 2 in, 2 out]
                n175 = property on="Test Slider" class="Slide (strict)"("Visible"=FALSE) -> ()  [unwired: 2 in, 2 out]
              }
              frame "White Balance  **" {
                n176 = Index Array(array=w301, index=1) -> (element=w302:cluster{string[]})
                n177 = call <vilib>:"NT Read String.vi"("Name"=w304) -> ("String"=w303:string)  [unwired: 9 in, 1 out]
                n178 = Unbundle(w302) -> (w299:string[])
                n179 = Match First String(2:w299, 3:w303) -> (0:w298:i32)  [unwired: 1 out]
                n180 = property on="Test Ring" class="Ring (strict)"("Value"=w298, "Strings []"=w299) -> ()  [unwired: 2 in, 2 out]
                n181 = property on="Test Ring" class="Ring (strict)"("Visible"=TRUE) -> ()  [unwired: 2 in, 2 out]
                n182 = property on="Test Slider" class="Slide (strict)"("Visible"=FALSE) -> ()  [unwired: 2 in, 2 out]
              }
              frame "Exposure  **" {
                n183 = Index Array(array=w310, index=2) -> (element=w311:cluster{string[]})
                n184 = call <vilib>:"NT Read String.vi"("Name"=w313) -> ("String"=w312:string)  [unwired: 9 in, 1 out]
                n185 = Unbundle(w311) -> (w307:string[])
                n186 = Match First String(2:w307, 3:w312) -> (0:w308:i32)  [unwired: 1 out]
                n187 = property on="Test Ring" class="Ring (strict)"("Value"=w308, "Strings []"=w307) -> ()  [unwired: 2 in, 2 out]
                n188 = property on="Test Ring" class="Ring (strict)"("Visible"=TRUE) -> ()  [unwired: 2 in, 2 out]
                n189 = property on="Test Slider" class="Slide (strict)"("Visible"=FALSE) -> ()  [unwired: 2 in, 2 out]
              }
              frame "Exposure Priority  **" {
                n190 = Index Array(array=w319, index=3) -> (element=w320:cluster{string[]})
                n191 = call <vilib>:"NT Read String.vi"("Name"=w322) -> ("String"=w321:string)  [unwired: 9 in, 1 out]
                n192 = Unbundle(w320) -> (w316:string[])
                n193 = Match First String(2:w316, 3:w321) -> (0:w317:i32)  [unwired: 1 out]
                n194 = property on="Test Ring" class="Ring (strict)"("Value"=w317, "Strings []"=w316) -> ()  [unwired: 2 in, 2 out]
                n195 = property on="Test Ring" class="Ring (strict)"("Visible"=TRUE) -> ()  [unwired: 2 in, 2 out]
                n196 = property on="Test Slider" class="Slide (strict)"("Visible"=FALSE) -> ()  [unwired: 2 in, 2 out]
              }
              frame "Color Enable  **" {
                n197 = Index Array(array=w328, index=4) -> (element=w329:cluster{string[]})
                n198 = call <vilib>:"NT Read String.vi"("Name"=w331) -> ("String"=w330:string)  [unwired: 9 in, 1 out]
                n199 = Unbundle(w329) -> (w325:string[])
                n200 = Match First String(2:w325, 3:w330) -> (0:w326:i32)  [unwired: 1 out]
                n201 = property on="Test Ring" class="Ring (strict)"("Value"=w326, "Strings []"=w325) -> ()  [unwired: 2 in, 2 out]
                n202 = property on="Test Ring" class="Ring (strict)"("Visible"=TRUE) -> ()  [unwired: 2 in, 2 out]
                n203 = property on="Test Slider" class="Slide (strict)"("Visible"=FALSE) -> ()  [unwired: 2 in, 2 out]
              }
              frame Default {
                n204 = property on="Test Ring" class="Ring (strict)"("Visible"=FALSE) -> ()  [unwired: 2 in, 2 out]
                n205 = property on="Test Slider" class="Slide (strict)"("Visible"=FALSE) -> ()  [unwired: 2 in, 2 out]
              }
              frame "Brightness  **", "Color Level  **", "Compression  **", "FPS  **", "Sharpness  **" {
                n206 = call <vilib>:"NT Read Number.vi"("Name"=w337) -> ("Numeric"=w336:dbl)  [unwired: 9 in, 1 out]
                n207 = local write "Test Slider"(w336) -> ()
                n208 = property on="Test Slider" class="Slide (strict)"("Visible"=TRUE, "Scale.Maximum"=100.0 ("Scale.Range:Maximum")) -> ()  [unwired: 2 in, 2 out]
                n209 = property on="Test Ring" class="Ring (strict)"("Visible"=FALSE) -> ()  [unwired: 2 in, 2 out]
              }
            }
          }
        }
        n210 = property on="Progress" class="Clust (strict)"("Visible"=FALSE) -> ()  [unwired: 2 in, 2 out]
      }
      event "Test Name": Mouse Enter {
        # "Populate the ring with the list of tests"
        n211 = event-data() -> ()  [unwired: 1 in, 1 out]
        n212 = call <vilib>:"NT Read String Array.vi"("Name"="/TestMode/TestList") -> ("String Array"=w345:string[])  [unwired: 9 in, 1 out]
        n213 = Build Array (concatenate)("Select the test to run...", w345) -> (w344:string[])
        n214 = property on="Test Name" class="Ring (strict)"("Strings []"=w344) -> ()  [unwired: 2 in, 2 out]
      }
      event "Test Name": Value Change {
        w347 = FALSE ("Visible")
        # "Tell the robot the test name to run"
        n215 = event-data() -> ("NewVal"=w351:u16)  [unwired: 1 in]
        n216 = property on="Test Name" class="Ring (strict)"() -> ("Strings []"=w352:string[])  [unwired: 2 in, 2 out]
        n217 = local write "Progress"(T6 {"Test Progress"=0, "Test Progress Text"=""} ("Progress")) -> ()
        n218 = Index Array(array=w352, index=w351) -> (element=w350:string)
        n219 = call <vilib>:"NT Write String.vi"("String"=w350, "Name"="/TestMode/TestName") -> ()  [unwired: 9 in, 1 out]
        n220 = property on="Progress" class="Clust (strict)"("Visible"=TRUE) -> ()  [unwired: 2 in, 2 out]
        n221 = property on="Motor" class="Clust (strict)"("Visible"=w347) -> ()  [unwired: 2 in, 2 out]
        n222 = property on="Test Slider" class="Slide (strict)"("Visible"=w347) -> ()  [unwired: 2 in, 2 out]
        n223 = property on="On/Off" class="Bool (strict)"("Visible"=w347) -> ()  [unwired: 2 in, 2 out]
        n224 = property on="Rev/Fwd" class="Clust (strict)"("Visible"=w347) -> ()  [unwired: 2 in, 2 out]
        n225 = property on="Test Ring" class="Ring (strict)"("Visible"=w347) -> ()  [unwired: 2 in, 2 out]
      }
      event "Select Auto": Mouse Enter {
        # "Populate the combo box with the list of autonomous options"
        n226 = event-data() -> ()  [unwired: 1 in, 1 out]
        n227 = call <vilib>:"NT Read String Array.vi"("Name"="Auto List") -> ("String Array"=w354:string[])  [unwired: 9 in, 1 out]
        n228 = property on="Select Auto" class="CmbBox"("Strings[]"=w354) -> ()  [unwired: 2 in, 2 out]
      }
      event "Select Auto": Value Change {
        # "User modified the Auto Selection. Write to NT variable so robot knows."
        n229 = event-data() -> ("NewVal"=w357:string)  [unwired: 1 in]
        n230 = call <vilib>:"NT Write String.vi"("String"=w357, "Name"="Auto Selector") -> ()  [unwired: 9 in, 1 out]
      }
      event "Command Selection": Value Change {
        # "Get the params and show in table"
        n231 = event-data() -> ("NewVal"=w363:i32)  [unwired: 1 in]
        n232 = property on="Command Selection" class="MCListbox (strict)"() -> ("ItemNames"=w361:string[][])  [unwired: 2 in, 2 out]
        n233 = call <vilib>:"WPI_DashboardUpdate Command Params.vi"("NewVal"=w363, "Commands"=w361, "Param Tbl"=w362) -> ()  [unwired: 8 in, 1 out]
      }
      event "Execute Command": Value Change {
        # "Started one, Unique ID holds\nresponse"
        n234 = event-data() -> ()  [unwired: 1 in, 1 out]
        n235 = property on="Command Selection" class="MCListbox (strict)"() -> ("ItemNames"=w374:string[][])  [unwired: 2 in, 2 out]
        n236 = Index Array(array=w374, index (row)="Command Selection", index (col)=0) -> (element=w372:string)
        n237 = call <vilib>:"Invoke Commands.vi"("Command Params"="Command Params", "Function Name"=w372) -> ("Params"=w368:u8, "Started"=w367:bool)  [unwired: 7 in, 1 out]
        n238 = Array Subset(array="Command Params", length (row)=w368) -> (w369:string[][])  [unwired: 3 in]
        n239 = Select(t="Executing" ("Cmd Status"), s=w367, f="" ("Cmd Status")) -> (s? t:f=→"Cmd Status":string)
      }
      event "Command Selection": Double Click {
        n240 = event-data() -> ("Row"=w382:i32)  [unwired: 1 in]
        n241 = property on="Command Selection" class="MCListbox (strict)"() -> ("ItemNames"=w385:string[][])  [unwired: 2 in, 2 out]
        n242 = local read "Command Params"() -> (w381:string[][])
        n243 = Index Array(array=w385, index (row)=w382, index (col)=0) -> (element=w383:string)
        n244 = call <vilib>:"Invoke Commands.vi"("Command Params"=w381, "Function Name"=w383) -> ("Params"=w380:u8, "Started"=w375:bool)  [unwired: 7 in, 1 out]
        n245 = Array Subset(array=w381, length (row)=w380) -> (w379:string[][])  [unwired: 3 in]
        n246 = Select(t="Executing" ("Cmd Status"), s=w375, f="" ("Cmd Status")) -> (s? t:f=w376:string)
        n247 = local write "Cmd Status"(w376) -> ()
      }
      event "CheckList": Double Click {
        # "Shift clears all"
        # "Update symbols on the listbox"
        n248 = event-data() -> ("PlatMods.Shift"=w387:bool, "Row"=w389:i32)  [unwired: 1 in]
        n249 = case shown="True" w387 {
          tunnel: w389 -> [w393 _]
          tunnel: 1 -> [w392 _]
          frame False {
            n250 = property on="CheckList" class="LstBox (strict)"() -> ("Item Symbols"=w391:i32[])  [unwired: 2 in, 2 out]
            n251 = Replace Array Subset(array=w391, new element=w392, index=w393) -> (w390:i32[])
            n252 = property on="CheckList" class="LstBox (strict)"("Item Symbols"=w390) -> ()  [unwired: 2 in, 2 out]
          }
          frame True {
            w394 = 0 ("Top Row")
            n253 = property on="CheckList" class="LstBox (strict)"() -> ("Number of Rows"=w396:u32)  [unwired: 2 in, 2 out]
            n254 = Initialize Array(0, w396) -> (w395:i32[])
            n255 = property on="CheckList" class="LstBox (strict)"("Top Row"=w394, "Value"=w394, "Item Symbols"=w395) -> ()  [unwired: 2 in, 2 out]
          }
        }
      }
      event "CheckList": Key Down {
        # "Update symbols on the listbox\nLeft and right keys check and uncheck"
        n256 = event-data() -> ("VKey"=w400:T19)  [unwired: 1 in]
        n257 = case shown="\"Left\", \"Right\"" w400 {
          selector: w400 -> [w405 _]
          tunnel: eventvkey."Left" ("VKey") -> [w403 _]
          frame "Left", "Right" {
            n258 = Equal?(x=w403, y=w405) -> (x = y?=w404:bool)
            n259 = Select(t=0, s=w404, f=1) -> (s? t:f=w406:i32)
            n260 = property on="CheckList" class="LstBox (strict)"() -> ("Item Symbols"=w409:i32[])  [unwired: 2 in, 2 out]
            n261 = Replace Array Subset(array=w409, new element=w406, index="CheckList") -> (w408:i32[])
            n262 = property on="CheckList" class="LstBox (strict)"("Item Symbols"=w408) -> ()  [unwired: 2 in, 2 out]
          }
          frame Default {
          }
        }
      }
      event "Motor.Enable": Value Change {
        # "When the test mode otor enable helper is set, update that\ntree row item's value"
        n263 = event-data() -> ("NewVal"=w415:bool)  [unwired: 1 in]
        n264 = Unbundle("Motor") -> ("Value"=w414:dbl)  [unwired: 1 out]
        n265 = Select(t=w414, s=w415, f=0.0) -> (s? t:f=w412:dbl)
        n266 = call <vilib>:"NT Write Number.vi"("Numeric"=w412, "Name"=w411) -> ()  [unwired: 9 in, 1 out]
      }
      event "Test Slider": Value Change {
        # "When the test mode slider helper is set, update that\ntree row item's value"
        n267 = event-data() -> ("NewVal"=w418:dbl)  [unwired: 1 in]
        n268 = call <vilib>:"NT Write Number.vi"("Numeric"=w418, "Name"=w419) -> ()  [unwired: 9 in, 1 out]
      }
      event "On/Off": Value Change {
        # "When the test mode on/off helper value is set, update that\ntree row item's value"
        n269 = event-data() -> ("NewVal"=w423:bool)  [unwired: 1 in]
        n270 = Boolean To (0,1)(Boolean=w423) -> (0, 1=w422:i16)
        n271 = call <vilib>:"NT Write Number.vi"("Numeric"=w422, "Name"=w421) -> ()  [unwired: 9 in, 1 out]
      }
      event "Rev/Fwd": Value Change {
        # "When the test mode helper value for relays is set, update that\ntree row item's value"
        n272 = event-data() -> ("NewVal.Forward"=w431:bool, "NewVal.Reverse"=w430:bool)  [unwired: 1 in]
        n273 = Boolean To (0,1)(Boolean=w431) -> (0, 1=w427:i16)
        n274 = Boolean To (0,1)(Boolean=w430) -> (0, 1=w429:i16)
        n275 = Negate(x=w429) -> (-x=w428:i16)
        n276 = Add(x=w427, y=w428) -> (x+y=w426:i16)
        n277 = call <vilib>:"NT Write Number.vi"("Numeric"=w426, "Name"=w425) -> ()  [unwired: 9 in, 1 out]
      }
      event "Test Ring": Value Change {
        # "When a test mode helper value is selected from the ring,\nset the tree item's variable to the string value"
        n278 = event-data() -> ("NewVal"=w435:u16)  [unwired: 1 in]
        n279 = property on="Test Ring" class="Ring (strict)"() -> ("Strings []"=w436:string[])  [unwired: 2 in, 2 out]
        n280 = Index Array(array=w436, index=w435) -> (element=w434:string)
        n281 = call <vilib>:"NT Write String.vi"("String"=w434, "Name"=w433) -> ()  [unwired: 9 in, 1 out]
      }
      event "Rec Mode": Value Change {
        # "Update globals for recording mode and path to read log from.\nClear when logging and let NetworkTables set path for vision to\nuse."
        n282 = event-data() -> ("NewVal"=w447:enum32{"Stop", "Record", "Playback"})  [unwired: 1 in]
        n283 = global write "WPI_DashboardLogging Global.vi" "Logging Filename"(path "") -> ()
        n284 = global write "WPI_DashboardLogging Global.vi" "Recording"(w447) -> ()
        n285 = case shown="\"Playback\"" w447 {
          tunnel: w446 -> [_ w449 w458]
          tunnel: [_ _ w457] -> w444
          tunnel: [_ _ w456] -> _
          tunnel: w442 -> [_ _ w454]
          tunnel: cluster{i32, i32} {-250, 170} -> [_ _ w453]
          tunnel: [_ _ T20 {"Image Size"=TRUE, "Image Type"=TRUE, "Pixel Value"=TRUE, "ROI Information"=TRUE, "Zoom Factor"=FALSE} ("Image Information Shown:All Elements")] -> w440
          tunnel: [_ _ TRUE ("Zoom Factor")] -> w439
          tunnel: w438 -> [_ _ w450]
          frame Default {
          }
          frame "Stop", "Record" {
            # "Place Window too"
            n286 = invoke class="VI" method="FP.Close"(reference=w449) -> (reference out=w448:refnum<vi>)  [unwired: 2 in, 2 out]
            n287 = invoke class="VI" method="Abort VI"(reference=w448) -> ()  [unwired: 2 in, 3 out]
          }
          frame "Playback" {
            n288 = call "Open Playback Panel.vi"("Offset"=w453, "DB VI Ref"=w454, "Playback in"=w458) -> ("Playback out"=w455:refnum<vi>)  [unwired: 8 in]
            n289 = register-events(w455, w450) -> (reference out=w457:refnum<event-registration>, error out=w456:errorcluster)  [unwired: 2 in]
          }
        }
        n290 = property on="Camera Image" class="ImageControl"("Image Information Shown"=w440, "Image Information Visible"=w439) -> ()  [unwired: 2 in, 2 out]
        n291 = call <vilib>:"WPI_DashboardNT Log FieldName Cache.vi"("Operation"=enum16{"Lookup/Add", "Index", "Clear"}."Clear") -> ()  [unwired: 8 in, 3 out]
      }
      event Panel Close {
        w460 = enum32{"Stop", "Record", "Playback"}."Stop" ("Rec Mode")
        # "Playback window has been closed, abort"
        n292 = event-data() -> ()  [unwired: 1 in, 4 out]
        n293 = local write "Rec Mode"(w460) -> ()
        n294 = global write "WPI_DashboardLogging Global.vi" "Recording"(w460) -> ()
      }
      event Panel Close {
        # "Abort playback window and ourself"
        n295 = event-data() -> ()  [unwired: 1 in, 4 out]
        n296 = invoke class="VI" method="FP.Close"(reference=w464) -> (reference out=w463:refnum<vi>)  [unwired: 2 in, 2 out]
        n297 = invoke class="VI" method="Abort VI"(reference=w463) -> (error out=w462:errorcluster)  [unwired: 2 in, 2 out]
        n298 = invoke class="VI" method="Abort VI"(error in=w462) -> ()  [unwired: 2 in, 3 out]
      }
      event User Event {
        n299 = event-data() -> ("IDs"=w471:cluster{"RPC field ID":u16, "Unique ID":u16}, "String"=w470:string)  [unwired: 1 in]
        n300 = Bundle("IDs"=w471, "String"=w470) -> (w469:T8)  [unwired: 1 in]
        n301 = call <vilib>:"Retrieve RPC Response.vi"("RPC Response"=w469) -> ("Output"=w467:string[][])  [unwired: 10 in]
        n302 = Build Array (concatenate)(w465, w467) -> (w466:string[][])
        n303 = local write "Command Params"(w466) -> ()
        n304 = local write "Cmd Status"("" ("Cmd Status")) -> ()
      }
      event "Tree": Double Click {
        n305 = event-data() -> ("PlatMods"=w475:T23, "Tag"=w474:string)  [unwired: 1 in]
        n306 = Unbundle(w475) -> ("Shift"=w473:bool)  [unwired: 4 out]
        n307 = Not(x=w473) -> (.not. x?=w472:bool)
        n308 = call <vilib>:"NT Update Persistence.vi"("Persistence"=w472, "Name"=w474) -> ()  [unwired: 9 in, 1 out]
      }
    }
  }
  n309 = while {
    tunnel: w64 -> [w478]
    i -> [w481]
    stop <- FALSE stop-if-true
    n310 = Wait (ms)(milliseconds to wait=u32 100) -> ()  [unwired: 1 out]
    n311 = case shown="\"Playback\"" "Rec Mode" {
      tunnel: w481 -> [_ _ w496]
      tunnel: [u32 2829099 ("Base Color") u32 11141120 ("Target Color") w485] -> w477
      frame "Stop", Default {
        # "Reset the color, extra updates don't cost much"
      }
      frame "Record" {
      }
      frame "Playback" {
        # "Playback"
        n312 = Quotient & Remainder(x=w496, y=u32 50 ("milliseconds to wait")) -> (x-y*floor(x/y)=w492:u32)  [unwired: 1 out]
        n313 = Divide(x=w492, y=u32 50 ("milliseconds to wait")) -> (x/y=w489:dbl)
        n314 = Multiply(x=6.283185307179586, y=w489) -> (x*y=w494:dbl)
        n315 = Sine(x=w494) -> (sin(x)=w493:dbl)
        n316 = Absolute Value(x=w493) -> (abs(x)=w486:dbl)
        n317 = call "Interpolate RGB Color.vi"("Proportion"=w486, "Target Color"=u32 30976, "Base Color"=u32 2829099) -> ("Result Color"=w485:u32)  [unwired: 8 in]
      }
    }
    n318 = property class="Pane"(reference=w478, "PaneColor"=w477) -> ()  [unwired: 1 in, 2 out]
  }
  n319 = local write "Dashboard Tab"(T2."Drive" ("Dashboard Tab")) -> ()
  n320 = property on="On/Off" class="Bool (strict)"("Visible"=w33) -> ()  [unwired: 2 in, 2 out]
  n321 = property on="Motor" class="Clust (strict)"("Visible"=w33) -> ()  [unwired: 2 in, 2 out]
  n322 = property on="Progress" class="Clust (strict)"("Visible"=w33) -> ()  [unwired: 2 in, 2 out]
  n323 = property on="Test Ring" class="Ring (strict)"("Visible"=w33) -> ()  [unwired: 2 in, 2 out]
  n324 = property on="Rev/Fwd" class="Clust (strict)"("Visible"=w33) -> ()  [unwired: 2 in, 2 out]
  n325 = while {
    tunnel: u16 1741 ("timeout ms (25000)") -> [w498]
    stop <- FALSE stop-if-true
    n326 = TCP Create Listener(10:w498) -> (0:w497:errorcluster, 3:w499:refnum<k5>)  [unwired: 4 in, 1 out]
    n327 = case shown="No Error" w497 {
      selector: w497 -> [w501 _]
      tunnel: w499 -> [w502 _]
      frame No Error {
        n328 = while {
          tunnel: w502 -> [w505]
          tunnel: w501 -> [w504]
          stop <- FALSE stop-if-true
          n329 = TCP Wait On Listener(8:w504, 11:w505) -> (0:w506:errorcluster, 4:w507:refnum<k5>)  [unwired: 2 in, 3 out]
          n330 = local write "TCP"(w507) -> ()
          n331 = case shown="No Error" w506 {
            frame No Error {
            }
            frame Error {
              n332 = Wait (ms)(milliseconds to wait=u32 1000) -> ()  [unwired: 1 out]
            }
          }
        }
      }
      frame Error {
        n333 = Wait (ms)(milliseconds to wait=u32 1000) -> ()  [unwired: 1 out]
      }
    }
  }
  n334 = local write "Command Selection"(u16 0 ("milliseconds to wait")) -> ()
  n335 = local write "Command Params"(string[][] [] ("Command Params")) -> ()
  n336 = global write "WPI_DashboardLogging Global.vi" "Recording"(w58) -> ()
  n337 = local write "Rec Mode"(w58) -> ()
  n338 = call <vilib>:"NT Write String.vi"("String"="Select Auto", "Name"="Auto Selector") -> ()  [unwired: 9 in, 1 out]
